vi "getTimeWithError.vi"(8 "error in (no error)":errorcluster) -> (0 "error out":errorcluster, 3 "seconds since 1Jan1904":timestamp)   [LabVIEW 2016, in "Instrument.Lockin.lvclass"]
uses:
  Instrument.Lockin.lvclass
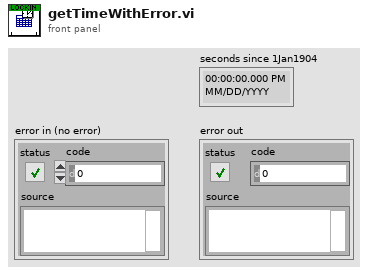
[diagram p1: front panel]
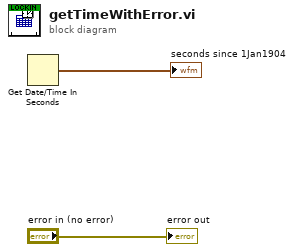
[diagram p0: block diagram]
diagram:
  n1 = Get Date/Time In Seconds() -> (seconds since 1Jan1904=→"seconds since 1Jan1904":timestamp)
  "error out" <- "error in (no error)"
